vi "XLP80_CAN_Main.vi"(7 "Function":string, 8 "error in":errorcluster, 10 "Input":variant) -> (0 "error out":errorcluster)   [LabVIEW 2021]
uses:
  <userlib>/PCAN Basic/Controls/CAN MSG Cluster.ctl
  <userlib>/PCAN Basic/Controls/Channel.ctl
  <userlib>/PCAN Basic/Controls/Parameter.ctl
  <userlib>/PCAN Basic/Controls/BaudrateEenum.ctl
  XLP80_Globals/XLP80_Globals_Status.vi
  XLP80_Globals/Globals_Settings_XLP80.vi
  <userlib>/PCAN Basic/VIs/Get Value/PCAN Get CHANNEL CONDITION.vi
  <userlib>/PCAN Basic/PCANBasic.lvlib
panel:
  in  "Signal Name":string[](array[string])
  in  "PEAK Data IN":T1[](array[typedef])=[{"ID"=84, "MSG type"=enum."STD", "LEN"=8, "DATA"=[2, 0, 0, 0, 0, 0, 0, 0]}] {"ID" format="%.0x"}
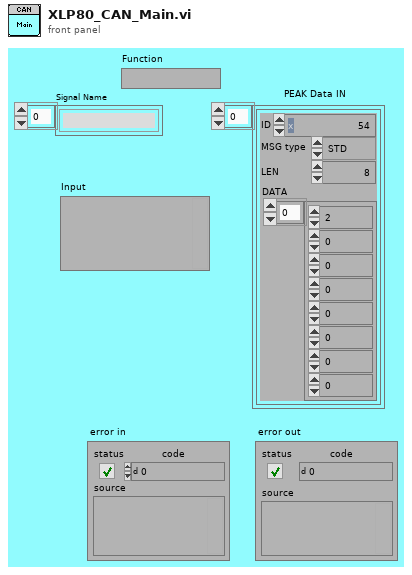
[diagram p1: front panel]
types:
  T1 = typedef "PCANBasic.lvlib/CAN MSG Cluster.ctl" = cluster{"ID":u32, "MSG type":enum8{"STD", "RTR", "XTD", "XTD RTR", "STATUS"}, "LEN":i8, "DATA":u8[]}
  T2 = typedef "XLP80_Action_TDefEnumControl.ctl" = enum16{"Testmode_A", "Testmode_B"}
  T3 = typedef "PCANBasic.lvlib/Channel.ctl" = enum16{"PCAN_NONEBUS", "not used1", "not used2", "not used3", "not used4", "not used5", "not used6", "not used7", "not used8", "not used9", "not used10", "not used11", "not used12", "not used13", "not used14", "not used15", "not used16", "not used17", "not used18", "not used19", "not used20", "not used21", "not used22", "not used23", "not used24", "not used25", "not used26", "not used27", "not used28", "not used29", "not used30", "not used31", "not used32", "PCAN_ISABUS1", "PCAN_ISABUS2", "PCAN_ISABUS3", "PCAN_ISABUS4", "PCAN_ISABUS5", "PCAN_ISABUS6", "PCAN_ISABUS7", "PCAN_ISABUS8", "not used41", "not used42", "not used43", "not used44", "not used45", "not used46", "not used47", "not used48", "PCAN_DNGBUS1", "not used50", "not used51", "not used52", "not used53", "not used54", "not used55", "not used56", "not used57", "not used58", "not used59", "not used60", "not used61", "not used62", "not used63", "not used64", "PCAN_PCIBUS1", "PCAN_PCIBUS2", "PCAN_PCIBUS3", "PCAN_PCIBUS4", "PCAN_PCIBUS5", "PCAN_PCIBUS6", "PCAN_PCIBUS7", "PCAN_PCIBUS8", "not used73", "not used74", "not used75", "not used76", "not used77", "not used78", "not used79", "not used80", "PCAN_USBBUS1", "PCAN_USBBUS2", "PCAN_USBBUS3", "PCAN_USBBUS4", "PCAN_USBBUS5", "PCAN_USBBUS6", "PCAN_USBBUS7", "PCAN_USBBUS8", "Not used89", "Not used90", "Not used91", "Not used92", "Not used93", "Not used94", "Not used95", "Not used96", "PCAN_PCCBUS1", "PCAN_PCCBUS2"}
  T4 = typedef "PCANBasic.lvlib/BaudrateEenum.ctl" = enum16{"CAN_Baud_1M", "CAN_Baud_800K", "CAN_BAUD_500K", "CAN_BAUD_250K", "CAN_BAUD_125K", "CAN_BAUD_100K", "CAN_BAUD_95K", "CAN_BAUD_83K", "CAN_BAUD_50K", "CAN_BAUD_47K", "CAN_BAUD_33K", "CAN_BAUD_20K", "CAN_BAUD_10K", "CAN_BAUD_5K", "User Baudrate"}
  T5 = typedef "PCANBasic.lvlib/Parameter.ctl" = enum16{"Not Available", "PCAN device number", "PCAN 5-volt power", "PCAN receive event", "PCAN message filter", "PCAN API version", "PCAN channel version", "PCAN bus-off auto reset", "PCAN listen-only", "PCAN log location", "PCAN log status", "PCAN log configure", "PCAN log text", "PCAN channel condition", "PCAN hardware name"}
  T6 = cluster{"Signal Name":string[], "Description":string[], "Unit":string[], "Default":dbl[], "Min":dbl[], "Max":dbl[], "Preconditions":bool[], "HV & Software":bool[], "Basis Funktion":bool[], "Power Management":bool[], "OperationMode":bool[], "Shutdown":bool[], "Alarm":bool[], "LogEnable":bool[]}
  T7 = cluster{"Signal Name":string[], "Description":string[], "Unit":string[], "Min":dbl[], "Max":dbl[], "HV & Software":bool[], "Basis Funktion":bool[], "Power Management":bool[], "OperationMode":bool[], "Shutdown":bool[], "Alarm":bool[], "LogEnable":bool[]}
  T8 = cluster{"Signal Name":string[], "Description":string[], "Unit":string[], "Min":dbl[], "Max":dbl[], "TestmodeA":bool[], "LogEnable":bool[]}
  T9 = cluster{"Signal Name":string[], "Description":string[], "Unit":string[], "Default":dbl[], "Min":dbl[], "Max":dbl[], "TestmodeA":bool[], "LogEnable":bool[]}
  T10 = typedef "PCANBasic.lvlib/Channel Availability.ctl" = enum16{"PCAN_CHANNEL_UNAVAILABLE", "PCAN_CHANNEL_AVAILABLE ", "PCAN_CHANNEL_OCCUPIED "}
  T11 = cluster{"CAN DBC":path, "Signal Name":string[], "Signal Name":string[]}
  T12 = typedef "PCANBasic.lvlib/Timestampbuffer.ctl" = cluster{"millis":u32, "millis_overflow":u16, "micros":u16}
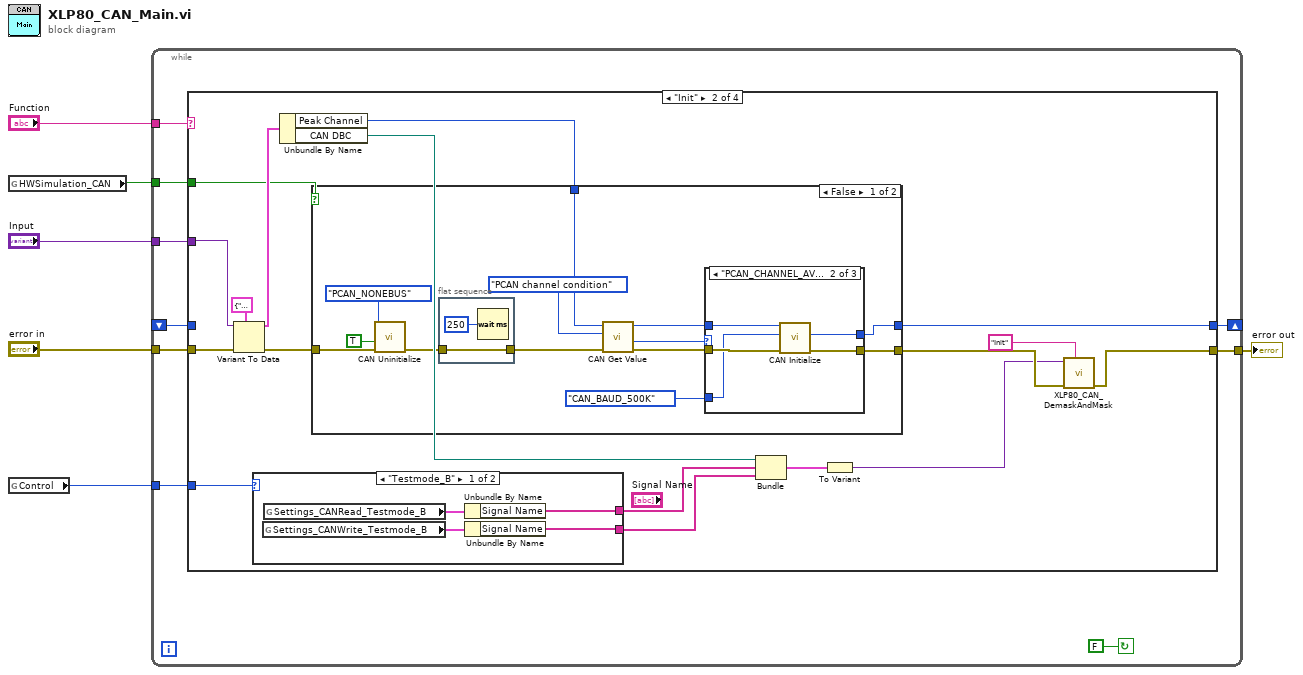
[diagram p0: block diagram]
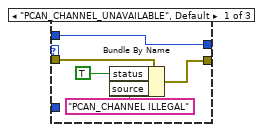
[diagram p3: hidden frame]
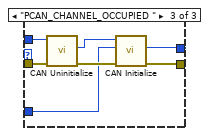
[diagram p4: hidden frame]
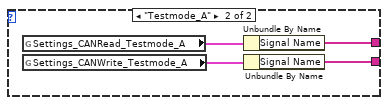
[diagram p6: hidden frame]
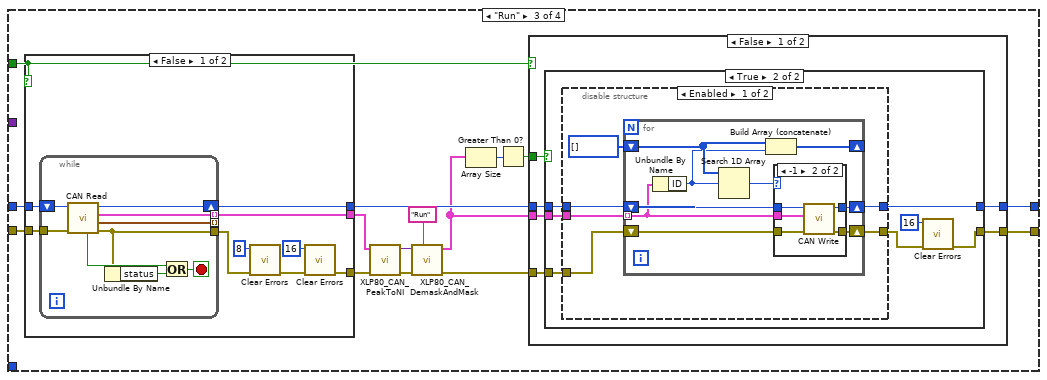
[diagram p7: hidden frame]
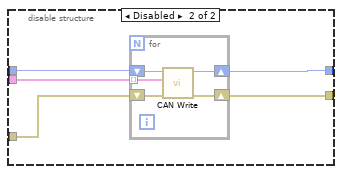
[diagram p10: hidden frame]
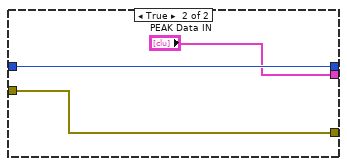
[diagram p12: hidden frame]
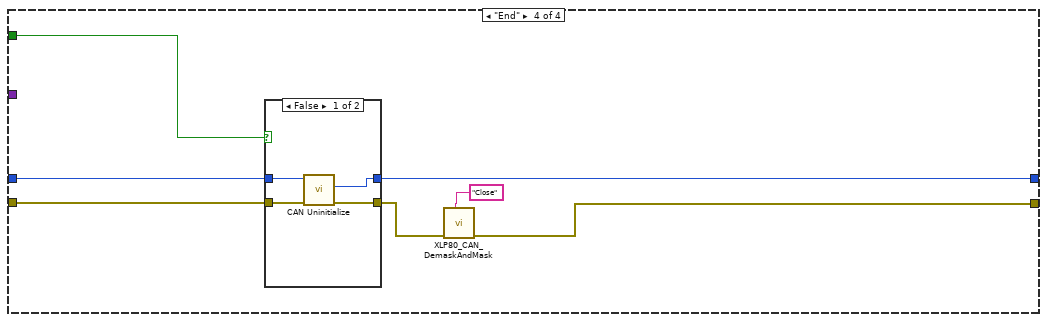
[diagram p13: hidden frame]
diagram:
  n1 = global read "Globals_Settings_XLP80.vi" "HWSimulation_CAN"() -> (w1:bool)
  n2 = global read "XLP80_Globals_Status.vi" "Control"() -> (w2:T2)
  n3 = while {
    tunnel: "error in" -> [w14]
    tunnel: "Function" -> [w13]
    shift-right: [w9] -> _
    shift-left: _ -> [w11]
    tunnel: [w12] -> w4
    tunnel: "Input" -> [w10]
    tunnel: w2 -> [w8]
    tunnel: w1 -> [w7]
    stop <- FALSE continue-if-true
    n4 = case shown="\"Init\"" w13 {
      tunnel: w14 -> [w16 w33 w90 w167]
      tunnel: [w16 w29 w87 w162] -> w12
      tunnel: w11 -> [w17 _ w89 w166]
      tunnel: w10 -> [_ w31 _ _]
      tunnel: [w17 w34 w88 w165] -> w9
      tunnel: w8 -> [_ w19 _ _]
      tunnel: w7 -> [_ w18 w79 w161]
      frame Default {
      }
      frame "Init" {
        n5 = Variant To Data(error in=w33, type=cluster{"Peak Channel":T3, "CAN DBC":path} {"Peak Channel"=enum."PCAN_NONEBUS", "CAN DBC"=path ""} ("output cluster"), Variant=w31) -> (data=w22:cluster{"Peak Channel":T3, "CAN DBC":path}, error out=w32:errorcluster)
        n6 = case shown="\"Testmode_B\"" w19 {
          tunnel: [w70 w74] -> w27
          tunnel: [w68 w72] -> w26
          frame "Testmode_B" {
            n7 = global read "Globals_Settings_XLP80.vi" "Settings_CANWrite_Testmode_B"() -> (w69:T6)
            n8 = global read "Globals_Settings_XLP80.vi" "Settings_CANRead_Testmode_B"() -> (w71:T7)
            n9 = Unbundle By Name(w71) -> ("Signal Name"=w70:string[])
            n10 = Unbundle By Name(w69) -> ("Signal Name"=w68:string[])
          }
          frame "Testmode_A" {
            n11 = global read "Globals_Settings_XLP80.vi" "Settings_CANRead_Testmode_A"() -> (w75:T8)
            n12 = global read "Globals_Settings_XLP80.vi" "Settings_CANWrite_Testmode_A"() -> (w73:T9)
            n13 = Unbundle By Name(w75) -> ("Signal Name"=w74:string[])
            n14 = Unbundle By Name(w73) -> ("Signal Name"=w72:string[])
          }
        }
        n15 = Unbundle By Name(w22) -> ("Peak Channel"=w21:T3, "CAN DBC"=w20:path)
        n16 = case shown="False" w18 {
          tunnel: [w38 _] -> w34
          tunnel: w32 -> [w37 w67]
          tunnel: [w36 w67] -> w30
          tunnel: w21 -> [w35 _]
          frame False {
            n17 = call <userlib>:"CAN Uninitialize.vi"("error in (no error)"=w37, "Ignore input error"=TRUE, "Channel"=Channel."PCAN_NONEBUS") -> ("error out"=w41:errorcluster)  [unwired: 6 in, 2 out]
            n18 = flat-sequence {
              tunnel: w41 -> [w48]
              tunnel: [w48] -> w40
              frame #0 {
                n19 = Wait (ms)(milliseconds to wait=u32 250) -> ()  [unwired: 1 out]
              }
            }
            n20 = call-poly <userlib>:"CAN Get Value.vi"("error in (no error)"=w40, "Parameter"=Parameter."PCAN channel condition", "Channel"=w35) -> ("error out"=w44:errorcluster, "Channel condition"=w45:T10, "Channel out"=w43:T3)  [unwired: 6 in]
            n21 = case shown="\"PCAN_CHANNEL_AVAILABLE \"" w45 {
              tunnel: [w50 w59 w61] -> w36
              tunnel: w43 -> [w54 w58 w65]
              tunnel: w44 -> [w53 w57 w66]
              tunnel: BaudrateEenum."CAN_BAUD_500K" ("BTR0BTR1") -> [_ w56 w62]
              tunnel: [w54 w55 w60] -> w38
              frame "PCAN_CHANNEL_UNAVAILABLE", Default {
                n22 = Bundle By Name(cluster=w53, "status"=TRUE, "source"="PCAN_CHANNEL ILLEGAL") -> (w50:errorcluster)
              }
              frame "PCAN_CHANNEL_AVAILABLE " {
                n23 = call <userlib>:"CAN Initialize.vi"("error in (no error)"=w57, "BTR0BTR1"=w56, "Channel"=w58) -> ("error out"=w59:errorcluster, "Channel out"=w55:T3)  [unwired: 6 in, 1 out]
              }
              frame "PCAN_CHANNEL_OCCUPIED " {
                n24 = call <userlib>:"CAN Uninitialize.vi"("error in (no error)"=w66, "Channel"=w65) -> ("error out"=w64:errorcluster, "Channel out"=w63:T3)  [unwired: 7 in, 1 out]
                n25 = call <userlib>:"CAN Initialize.vi"("error in (no error)"=w64, "BTR0BTR1"=w62, "Channel"=w63) -> ("error out"=w61:errorcluster, "Channel out"=w60:T3)  [unwired: 6 in, 1 out]
              }
            }
          }
          frame True {
          }
        }
        n26 = Bundle("CAN DBC"=w20, "Signal Name"=w27, "Signal Name"=w26) -> (w25:T11)  [unwired: 1 in]
        n27 = To Variant(anything=w25) -> (Variant=w24:variant)
        n28 = call "XLP80_CAN_DemaskAndMask.vi"("Function"="Init", "err in"=w30, "Variant"=w24) -> ("error out"=w29:errorcluster)  [unwired: 7 in, 1 out]
      }
      frame "Run" {
        n29 = case shown="False" w79 {
          tunnel: w90 -> [w148 w158]
          tunnel: w89 -> [w147 w160]
          tunnel: [w140 w158] -> w85
          tunnel: [w144 "PEAK Data IN"] -> w77
          tunnel: [w143 w160] -> w82
          frame False {
            n30 = while {
              tunnel: w148 -> [w155]
              tunnel: [w153] -> _ mode=indexing
              tunnel: [w154] -> w144 mode=indexing
              shift-right: [w149] -> w143
              shift-left: w147 -> [w152]
              tunnel: [w150] -> w146
              stop <- w157 stop-if-true
              n31 = call <userlib>:"CAN Read.vi"("error in (no error)"=w155, "Channel"=w152) -> ("error out"=w150:errorcluster, "TimestampBuffer out"=w153:T12, "CAN_Message out"=w154:T1, "Channel out"=w149:T3, "rcv queue empty"=w151:bool)  [unwired: 5 in]
              n32 = Unbundle By Name(w150) -> ("status"=w156:bool)
              n33 = Or(x=w151, y=w156) -> (x .or. y?=w157:bool)
            }
            n34 = call <vilib>:"Clear Errors.vi"("error in (no error)"=w146, "specific error code to clear (0: all)"=8) -> ("error out"=w141:errorcluster)  [unwired: 4 in, 1 out]
            n35 = call <vilib>:"Clear Errors.vi"("error in (no error)"=w141, "specific error code to clear (0: all)"=16) -> ("error out"=w140:errorcluster)  [unwired: 4 in, 1 out]
          }
          frame True {
          }
        }
        n36 = call "XLP80_CAN_PeakToNI.vi"("error in"=w85, "PEAK CANData Read"=w77) -> ("error out"=w84:errorcluster, "NI Data OUT"=w83:variant)  [unwired: 8 in]
        n37 = call "XLP80_CAN_DemaskAndMask.vi"("Function"="Run", "err in"=w84, "Variant"=w83) -> ("error out"=w76:errorcluster, "CANData Write"=w78:T1[])  [unwired: 7 in]
        n38 = Array Size(array=w78) -> (size(s)=w81:i32)
        n39 = Greater Than 0?(x=w81) -> (x > 0?=w80:bool)
        n40 = case shown="False" w79 {
          tunnel: [w96 w138] -> w88
          tunnel: [w95 w139] -> w87
          tunnel: w82 -> [w94 w138]
          tunnel: w76 -> [w93 w139]
          tunnel: w80 -> [w91 _]
          tunnel: w78 -> [w92 _]
          frame False {
            n41 = case shown="True" w91 {
              tunnel: w94 -> [w98 w105]
              tunnel: w93 -> [w97 w104]
              tunnel: [w98 w103] -> w96
              tunnel: [w97 w99] -> w95
              tunnel: w92 -> [_ w102]
              frame False {
              }
              frame True {
                n42 = disable-structure shown="Enabled" {
                  disable-tunnel: w105 -> [w111 w132]
                  disable-tunnel: w104 -> [w110 w131]
                  disable-tunnel: [w109 w130] -> w103
                  disable-tunnel: [w108 w129] -> w100
                  disable-tunnel: w102 -> [w107 w128]
                  frame Enabled {
                    n43 = for {
                      shift-right: [w119] -> w108
                      shift-left: w110 -> [w120]
                      tunnel: w107 -> [w116] mode=indexing
                      shift-right: [w117] -> w109
                      shift-left: w111 -> [w118]
                      shift-right: [w115] -> _
                      shift-left: u32[] [] -> [w114]
                      n44 = Unbundle By Name(w116) -> ("ID"=w113:u32)
                      n45 = Search 1D Array(1D array=w114, element=w113) -> (index of element=w112:i32)  [unwired: 1 in]
                      n46 = Build Array (concatenate)(w114, w113) -> (w115:u32[])
                      n47 = case shown="-1" w112 {
                        tunnel: w120 -> [w121 w127]
                        tunnel: [w121 w126] -> w119
                        tunnel: w118 -> [w122 w125]
                        tunnel: [w122 w124] -> w117
                        tunnel: w116 -> [_ w123]
                        frame Default {
                        }
                        frame -1 {
                          n48 = call <userlib>:"CAN Write.vi"("error in (no error)"=w127, "CAN_Message"=w123, "Channel"=w125) -> ("error out"=w126:errorcluster, "Channel out"=w124:T3)  [unwired: 7 in]
                        }
                      }
                    }
                  }
                  frame Disabled {
                    n49 = for {
                      shift-right: [w136] -> w129
                      shift-left: w131 -> [w137]
                      tunnel: w128 -> [w133] mode=indexing
                      shift-right: [w134] -> w130
                      shift-left: w132 -> [w135]
                      n50 = call <userlib>:"CAN Write.vi"("error in (no error)"=w137, "CAN_Message"=w133, "Channel"=w135) -> ("error out"=w136:errorcluster, "Channel out"=w134:T3)  [unwired: 7 in]
                    }
                  }
                }
                n51 = call <vilib>:"Clear Errors.vi"("error in (no error)"=w100, "specific error code to clear (0: all)"=16) -> ("error out"=w99:errorcluster)  [unwired: 4 in, 1 out]
              }
            }
          }
          frame True {
          }
        }
      }
      frame "End" {
        n52 = case shown="False" w161 {
          tunnel: w167 -> [w171 w172]
          tunnel: w166 -> [w170 w173]
          tunnel: [w169 w173] -> w165
          tunnel: [w168 w172] -> w163
          frame False {
            n53 = call <userlib>:"CAN Uninitialize.vi"("error in (no error)"=w171, "Channel"=w170) -> ("error out"=w168:errorcluster, "Channel out"=w169:T3)  [unwired: 7 in, 1 out]
          }
          frame True {
          }
        }
        n54 = call "XLP80_CAN_DemaskAndMask.vi"("Function"="Close", "err in"=w163) -> ("error out"=w162:errorcluster)  [unwired: 8 in, 1 out]
      }
    }
  }
  "error out" <- w4
